vi "Simple Global for Marker Options.vi"() -> ()   [LabVIEW 2015]
uses:
  MarkerOptions.ctl
  subVIs/MarkersDVRType.ctl
  markerType.ctl
panel:
  out "markers":T1[](array[typedef])
  in  "Options":T3={"Color"=16723218, "pen"={"Width"=2, "Style"=enum."Solid"}, "font"={"Font Name"="Arial", "Size"=14, "Strikeout?"=FALSE, "Italic?"=FALSE, "Underline?"=FALSE, "Outline?"=FALSE, "Shadow?"=FALSE, "Bold?"=FALSE, "FontColor"=6908265}, "caption"="Click to set a point marker"}
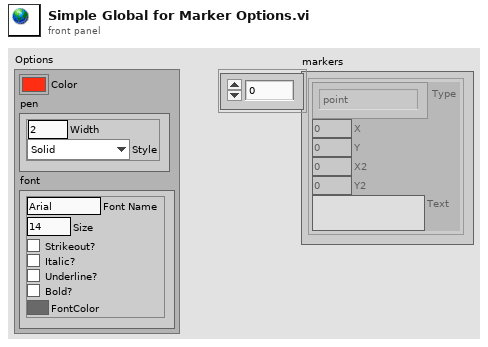
[diagram p1: front panel]
types:
  T1 = typedef "MarkersDVRType.ctl" = cluster{"Type":T2, "X":dbl, "Y":dbl, "X2":dbl, "Y2":dbl, "Text":string}
  T2 = typedef "markerType.ctl" = enum16{"point", "arrow", "horiz", "vert", "vert range", "horiz range", "box"}
  T3 = typedef "MarkerOptions.ctl" = cluster{"Color":u32, "pen":cluster{"Width":u16, "Style":enum32{"Solid", "Dash", "Dot", "DashDot", "DashDotDot"}}, "font":cluster{"Font Name":string, "Size":i16, "Strikeout?":bool, "Italic?":bool, "Underline?":bool, "Outline?":bool, "Shadow?":bool, "Bold?":bool, "FontColor":u32}, "caption":string}
diagram:
